vi "Set Elevator Speed.vi"(10 "Buttons":T1) -> (3 "Elevator Speed":dbl)   [LabVIEW 2011]
uses:
  <vilib>/Rock Robotics/WPI/Joystick/WPI_JoystickButtonState.ctl
  Robot Global Data.vi
panel:
  out "number":u32
  in  "Elevator Setting":dbl(slide)=0.9818181818181818 scale=0.0..1.0
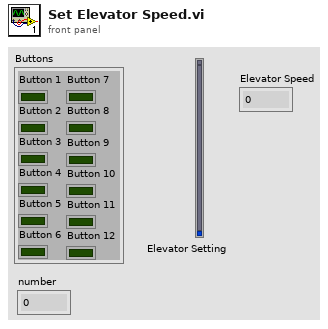
[diagram p1: front panel]
types:
  T1 = typedef "WPI_JoystickButtonState.ctl" = cluster{"Button 1":bool, "Button 2":bool, "Button 3":bool, "Button 4":bool, "Button 5":bool, "Button 6":bool, "Button 7":bool, "Button 8":bool, "Button 9":bool, "Button 10":bool, "Button 11":bool, "Button 12":bool}
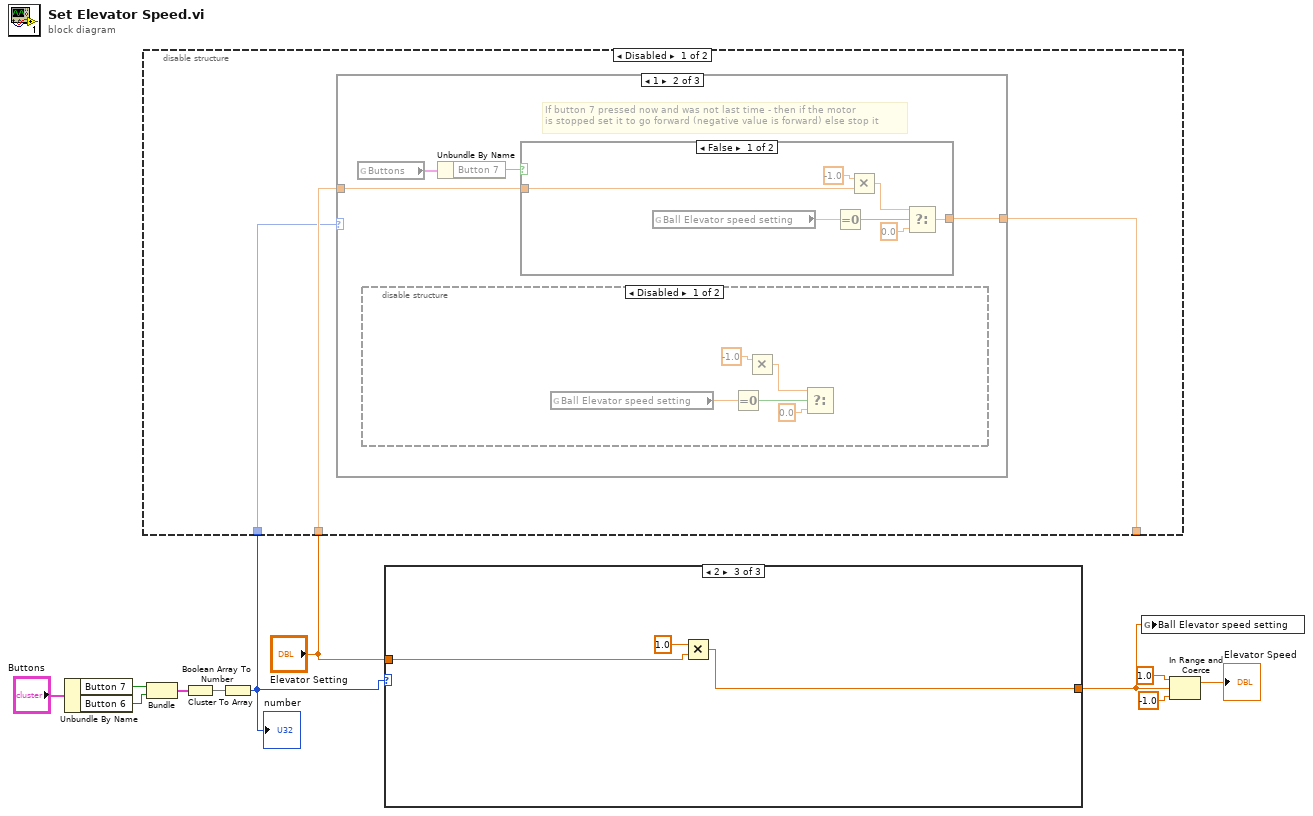
[diagram p0: block diagram]
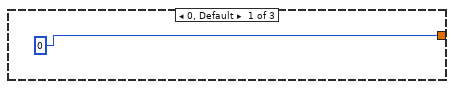
[diagram p2: hidden frame]
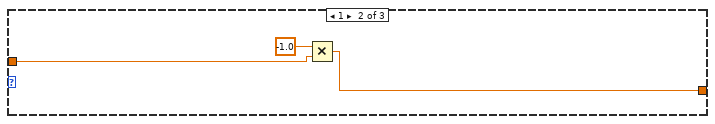
[diagram p3: hidden frame]
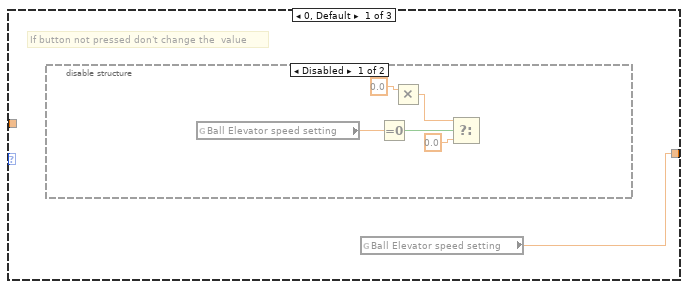
[diagram p4: hidden frame]
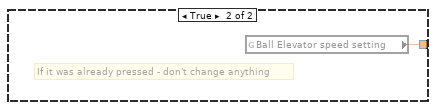
[diagram p7: hidden frame]
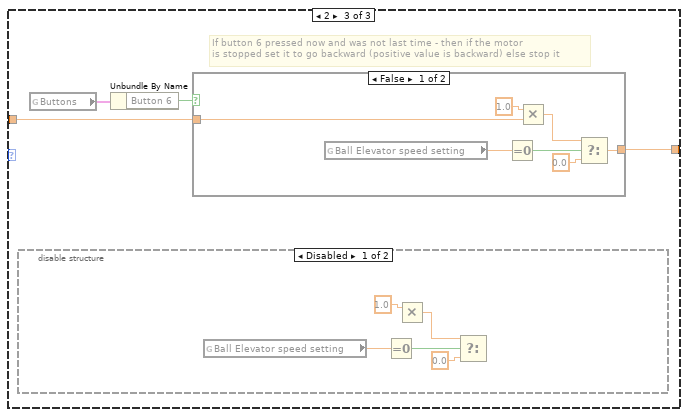
[diagram p8: hidden frame]
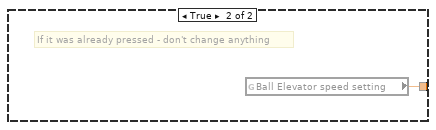
[diagram p10: hidden frame]
diagram:
  n1 = Unbundle By Name("Buttons") -> ("Button 7"=w7:bool, "Button 6"=w6:bool)
  n2 = Bundle("Button 7"=w7, "Button 6"=w6) -> (w5:cluster{"Button 7":bool, "Button 6":bool})  [unwired: 1 in]
  n3 = Cluster To Array(cluster=w5) -> (array=w4:bool[])
  n4 = Boolean Array To Number(Boolean array=w4) -> (number=w3:u32)
  "number" <- w3
  n5 = disable-structure shown="Disabled" {
    disable-tunnel: "Elevator Setting" -> [w14 _]
    disable-tunnel: w3 -> [w13 _]
    disable-tunnel: [w12 _] -> _
    frame Disabled {
      n6 = case shown="1" w13 {
        tunnel: [w15 w23 w42] -> w12
        tunnel: w14 -> [_ w26 w45]
        frame 0, Default {
          # "If button not pressed don't change the  value"
          n7 = disable-structure shown="Disabled" {
            frame Disabled {
              n8 = global read "Robot Global Data.vi" "Ball Elevator speed setting"() -> (w21:dbl)
              n9 = Equal To 0?(x=w21) -> (x = 0?=w22:bool)
              n10 = Multiply(x=0.0) -> (y=w17:dbl, x*y=w18:dbl)
              n11 = Select(t=w18, s=w22, f=0.0) -> (s? t:f=w16:dbl)
            }
            frame Enabled {
            }
          }
          n12 = global read "Robot Global Data.vi" "Ball Elevator speed setting"() -> (w15:dbl)
        }
        frame 1 {
          # "If button 7 pressed now and was not last time - then if the motor \nis stopped set it to go forward (negative value is forward) else stop it"
          n13 = global read "Robot Global Data.vi" "Buttons"() -> (w25:T1)
          n14 = disable-structure shown="Disabled" {
            frame Disabled {
              n15 = global read "Robot Global Data.vi" "Ball Elevator speed setting"() -> (w32:dbl)
              n16 = Equal To 0?(x=w32) -> (x = 0?=w33:bool)
              n17 = Multiply(x=-1.0) -> (y=w27:dbl, x*y=w29:dbl)
              n18 = Select(t=w29, s=w33, f=0.0) -> (s? t:f=w28:dbl)
            }
            frame Enabled {
            }
          }
          n19 = Unbundle By Name(w25) -> ("Button 7"=w24:bool)
          n20 = case shown="False" w24 {
            tunnel: [w37 w41] -> w23
            tunnel: w26 -> [w36 _]
            frame False {
              n21 = global read "Robot Global Data.vi" "Ball Elevator speed setting"() -> (w39:dbl)
              n22 = Equal To 0?(x=w39) -> (x = 0?=w40:bool)
              n23 = Multiply(x=-1.0, y=w36) -> (x*y=w34:dbl)
              n24 = Select(t=w34, s=w40, f=0.0) -> (s? t:f=w37:dbl)
            }
            frame True {
              # "If it was already pressed - don't change anything"
              n25 = global read "Robot Global Data.vi" "Ball Elevator speed setting"() -> (w41:dbl)
            }
          }
        }
        frame 2 {
          # "If button 6 pressed now and was not last time - then if the motor \nis stopped set it to go backward (positive value is backward) else stop it"
          n26 = disable-structure shown="Disabled" {
            frame Disabled {
              n27 = global read "Robot Global Data.vi" "Ball Elevator speed setting"() -> (w51:dbl)
              n28 = Equal To 0?(x=w51) -> (x = 0?=w52:bool)
              n29 = Multiply(x=1.0) -> (y=w46:dbl, x*y=w48:dbl)
              n30 = Select(t=w48, s=w52, f=0.0) -> (s? t:f=w47:dbl)
            }
            frame Enabled {
            }
          }
          n31 = global read "Robot Global Data.vi" "Buttons"() -> (w44:T1)
          n32 = Unbundle By Name(w44) -> ("Button 6"=w43:bool)
          n33 = case shown="False" w43 {
            tunnel: [w56 w60] -> w42
            tunnel: w45 -> [w55 _]
            frame False {
              n34 = global read "Robot Global Data.vi" "Ball Elevator speed setting"() -> (w58:dbl)
              n35 = Equal To 0?(x=w58) -> (x = 0?=w59:bool)
              n36 = Multiply(x=1.0, y=w55) -> (x*y=w53:dbl)
              n37 = Select(t=w53, s=w59, f=0.0) -> (s? t:f=w56:dbl)
            }
            frame True {
              # "If it was already pressed - don't change anything"
              n38 = global read "Robot Global Data.vi" "Ball Elevator speed setting"() -> (w60:dbl)
            }
          }
        }
      }
    }
    frame Enabled {
    }
  }
  n39 = case shown="2" w3 {
    tunnel: [0 w64 w67] -> w2
    tunnel: "Elevator Setting" -> [_ w62 w65]
    frame 0, Default {
    }
    frame 1 {
      n40 = Multiply(x=-1.0, y=w62) -> (x*y=w64:dbl)
    }
    frame 2 {
      n41 = Multiply(x=1.0, y=w65) -> (x*y=w67:dbl)
    }
  }
  n42 = global write "Robot Global Data.vi" "Ball Elevator speed setting"(w2) -> ()
  n43 = In Range and Coerce(upper limit=1.0, x=w2, lower limit=-1.0) -> (coerced(x)=→"Elevator Speed":dbl)  [unwired: 1 out]
